vi "Setting_E3632A.vi"(0 "Instrument In":refnum<visa-resource-name>, 2 "Set Out Voltage":dbl format="%.3g", 3 "Current Limit":dbl min=0.0 max=25.0 step=1.0 format="%.4f", 4 "Over Voltage Limit":dbl=61.0 min=0.0 max=151.0 step=0.001 format="%.3f", 5 "error in (no error)":errorcluster, 6 "Ring":u16(ring) items=["Disable", "Enable"]) -> (14 "Instrument Out":refnum<visa-resource-name>, 19 "error out":errorcluster)   [LabVIEW 2023]
uses:
  <instrlib>/Agilent E363X Series/Agilent E363X Series.lvlib
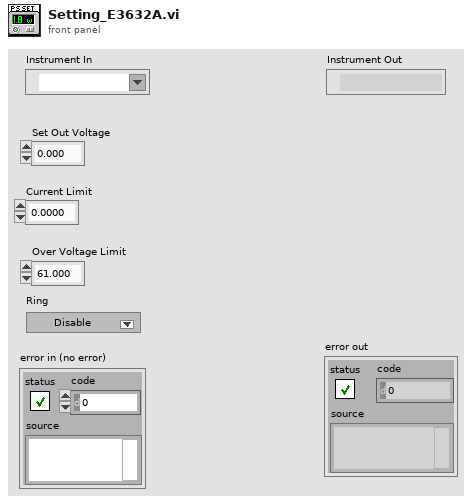
[diagram p1: front panel]
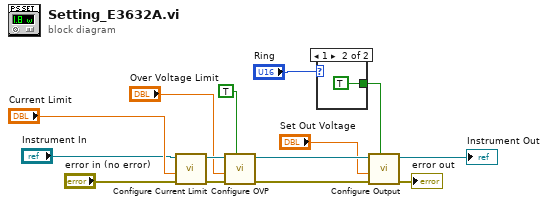
[diagram p0: block diagram]
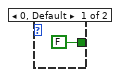
[diagram p2: hidden frame]
diagram:
  n1 = call <instrlib>:"Configure Current Limit.vi"("error in (no error)"="error in (no error)", "Current Limit (0.0 A)"="Current Limit", "VISA resource name"="Instrument In") -> ("error out"=w12:errorcluster, "VISA resource name out"=w13:refnum<visa-resource-name>)  [unwired: 7 in]
  n2 = call <instrlib>:"Configure OVP.vi"("Enable OVP (T: Enable)"=TRUE, "error in (no error)"=w12, "Voltage Limit (0.0 V)"="Over Voltage Limit", "VISA resource name"=w13) -> ("error out"=w8:errorcluster, "VISA resource name out"=w9:refnum<visa-resource-name>)  [unwired: 6 in]
  n3 = case shown="1" "Ring" {
    tunnel: [FALSE TRUE] -> w4
    frame 0, Default {
    }
    frame 1 {
    }
  }
  n4 = call <instrlib>:"Configure Output.vi"("Enable Output (T: Enable)"=w4, "error in (no error)"=w8, "Voltage Level (0.0 V)"="Set Out Voltage", "VISA resource name"=w9) -> ("error out"=→"error out":errorcluster, "VISA resource name out"=→"Instrument Out":refnum<visa-resource-name>)  [unwired: 6 in]
